vi "client.vi"() -> ()   [LabVIEW 2021]
panel:
  in  "Tab Control":T1(tab)
  in  "Indirizzo IP":string
  in  "f_start (Hz)":string
  in  "f_stop (Hz)":string
  in  "Step di frequenza (Hz)":string
  in  "Ampiezza (Vpp)":string
  in  "Password":string
  in  "?":bool
  out "Status misure":string
  in  "Porta":u16
  out "Trovata":bool
  out "Frequenza a -3dB (Hz)":string
  out "XY Graph":cluster{dbl[], dbl[]}(graph)
  # "SWEEP IN FREQUENZA"
  # "Università degli studi di Cassino e del Lazio Meridionale - Sistemi di Misura Distribuiti\nProf. Domenico Capriglione\nStudenti: Federico Coviello, Lorena De Simone, Giustino Marino, Giulio Russo"
  # "Istruzioni per l'uso"
  # "1. Inserire nel Pannello di controllo i parametri dello sweep in frequenza:\n- Frequenza di start\n- Frequenza di stop\n- Step in frequenza\n- Ampiezza\n- Porta (il Server risponde sulla porta 1001)\n\n2. Inserire la Password e, successivamente, iniziare le misure cliccando sul bottone \"INIZIO MISURE\"\n\n3. I risultati verranno riportati sul pannello \"Display\""
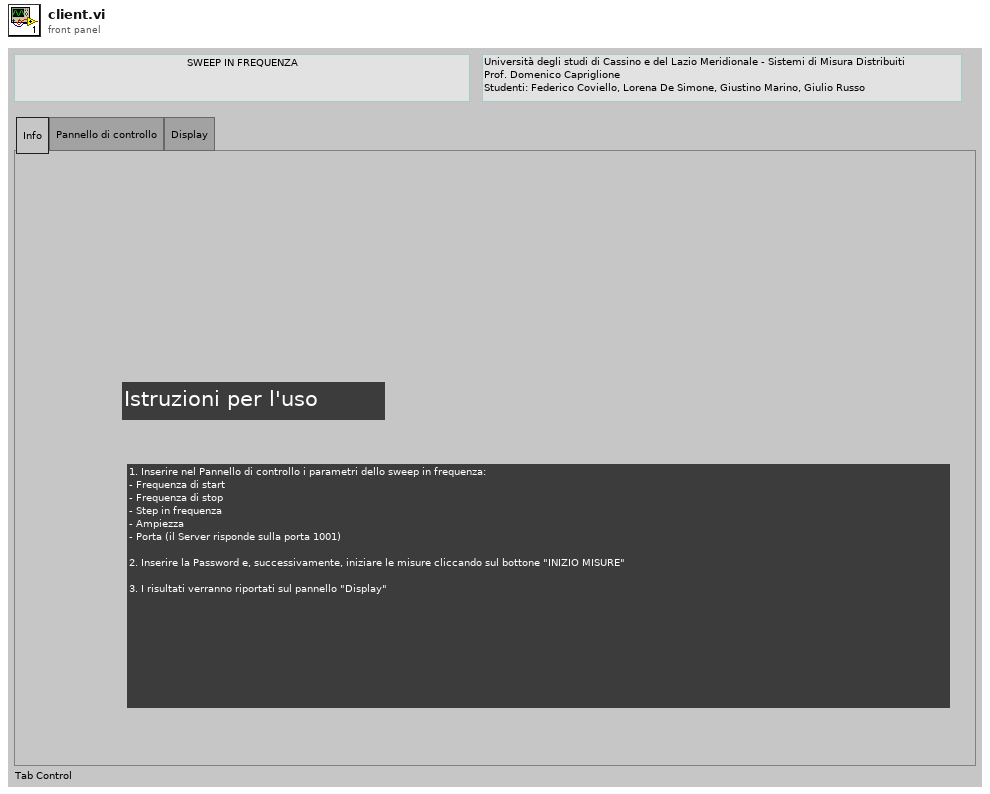
[diagram p1: front panel]
types:
  T1 = enum32{"Info", "Pannello di controllo", "Display"}
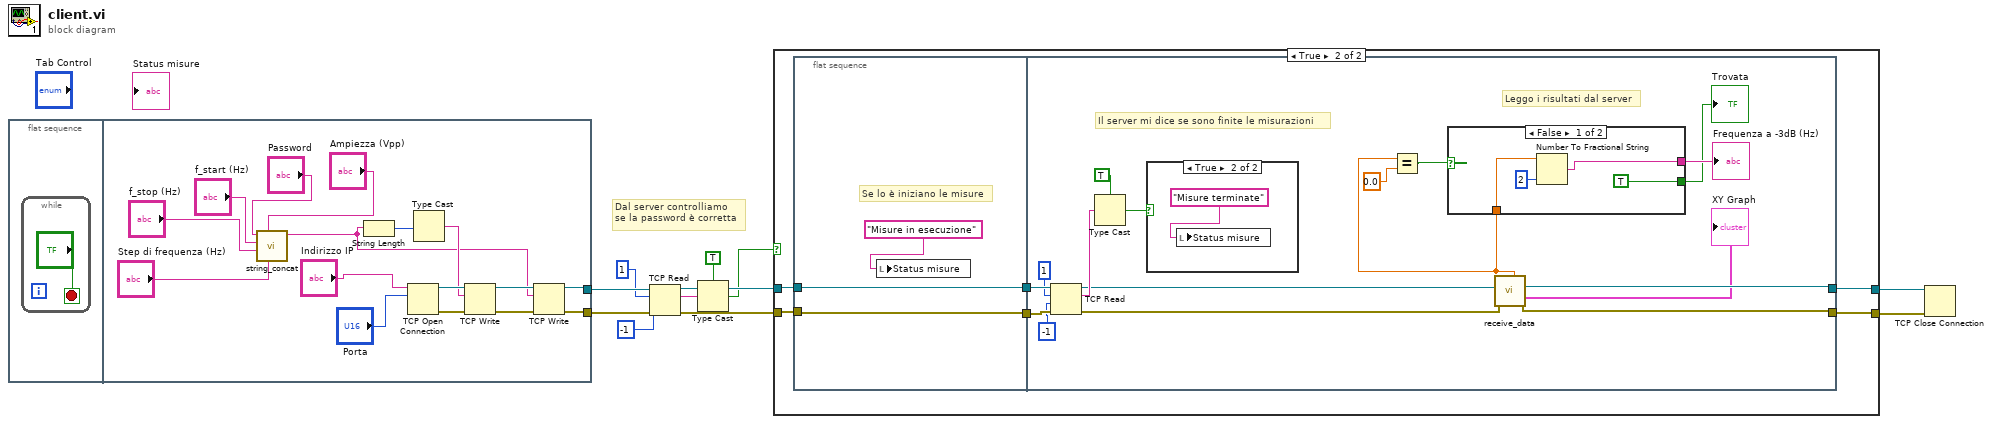
[diagram p0: block diagram]
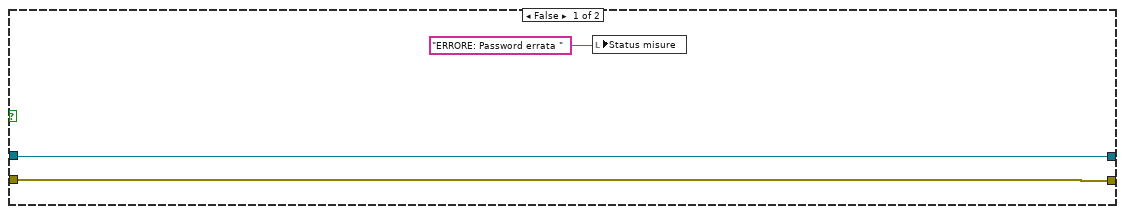
[diagram p2: hidden frame]
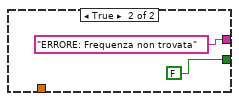
[diagram p3: hidden frame]
diagram:
  # "Dal server controlliamo\nse la password è corretta"
  n1 = flat-sequence {
    tunnel: [w15] -> w10
    tunnel: [w14] -> w11
    frame #0 {
      n2 = while {
        stop <- "?" stop-if-true
      }
    }
    frame #1 {
      n3 = call "string_concat.vi"("Step di frequenza (Hz)"="Step di frequenza (Hz)", "Ampiezza (Vpp)"="Ampiezza (Vpp)", "f_stop (Hz)"="f_stop (Hz)", "f_start (Hz)"="f_start (Hz)", "Password"="Password") -> ("Comando concatenato"=w18:string)  [unwired: 6 in]
      n4 = String Length(string=w18) -> (length=w23:i32)
      n5 = TCP Open Connection(address="Indirizzo IP", remote port or service name="Porta") -> (connection ID=w27:refnum<k5>, error out=w25:errorcluster)  [unwired: 3 in]
      n6 = Type Cast(x=w23) -> (*(type *) &x=w22:string)  [unwired: 1 in]
      n7 = TCP Write(connection ID=w27, data in=w22, error in (no error)=w25) -> (connection ID out=w26:refnum<k5>, error out=w24:errorcluster)  [unwired: 1 in, 1 out]
      n8 = TCP Write(connection ID=w26, data in=w18, error in (no error)=w24) -> (connection ID out=w14:refnum<k5>, error out=w15:errorcluster)  [unwired: 1 in, 1 out]
    }
  }
  n9 = TCP Read(connection ID=w11, bytes to read=1, error in (no error)=w10, 9:-1 ("timeout ms (25000)")) -> (connection ID out=w8:refnum<k5>, data out=w7:string, error out=w9:errorcluster)  [unwired: 1 in]
  n10 = Type Cast(type=TRUE, x=w7) -> (*(type *) &x=w5:bool)
  n11 = case shown="True" w5 {
    tunnel: w9 -> [w29 w35]
    tunnel: w8 -> [w30 w37]
    tunnel: [w30 w32] -> w3
    tunnel: [w29 w33] -> w4
    frame False {
      n12 = local write "Status misure"("ERRORE: Password errata ") -> ()
    }
    frame True {
      n13 = flat-sequence {
        tunnel: w37 -> [w40]
        tunnel: [w40] -> w36
        tunnel: w35 -> [w39]
        tunnel: [w39] -> w34
        tunnel: w36 -> [w56]
        tunnel: w34 -> [w55]
        tunnel: [w50] -> w33
        tunnel: [w49] -> w32
        frame #0 {
          # "Se lo è iniziano le misure"
          n14 = local write "Status misure"("Misure in esecuzione") -> ()
        }
        frame #1 {
          # "Leggo i risultati dal server"
          # "Il server mi dice se sono finite le misurazioni"
          n15 = TCP Read(connection ID=w56, bytes to read=1, error in (no error)=w55, 9:-1 ("timeout ms (25000)")) -> (connection ID out=w47:refnum<k5>, data out=w57:string, error out=w48:errorcluster)  [unwired: 1 in]
          n16 = Type Cast(type=TRUE, x=w57) -> (*(type *) &x=w54:bool)
          n17 = case shown="True" w54 {
            frame False {
            }
            frame True {
              n18 = local write "Status misure"("Misure terminate") -> ()
            }
          }
          n19 = call "receive_data.vi"("error in (no error)"=w48, "TCP Network Connection in"=w47) -> ("error out"=w50:errorcluster, "XY Graph"=→"XY Graph":cluster{dbl[], dbl[]}, "TCP Network Connection out"=w49:refnum<k5>, "Frequenza -3dB"=w42:dbl)  [unwired: 4 in, 2 out]
          n20 = Equal?(x=w42, y=0.0) -> (x = y?=w44:bool)
          n21 = case shown="False" w44 {
            tunnel: [w59 "ERRORE: Frequenza non trovata" ("Frequenza a -3dB")] -> w43
            tunnel: w42 -> [w61 _]
            tunnel: [TRUE FALSE] -> w41
            frame False {
              n22 = Number To Fractional String(number=w61, precision (6)=i16 2) -> (F-format string=w59:string)  [unwired: 2 in]
            }
            frame True {
            }
          }
          "Frequenza a -3dB (Hz)" <- w43
          "Trovata" <- w41
        }
      }
    }
  }
  n23 = TCP Close Connection(connection ID=w3, error in (no error)=w4) -> ()  [unwired: 1 in, 2 out]
